vi "2010 Connection Lookup Tests.vi"(8 "error in":errorcluster) -> (0 "error out":errorcluster)   [LabVIEW 2020, in "Test_Routing Templates.lvlib"]
uses:
  Test_Routing Templates.lvlib
  <vilib>/addons/_JKI Toolkits/Caraya/classes/Test/Test.lvclass
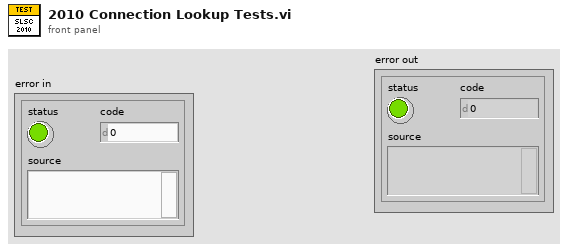
[diagram p1: front panel]
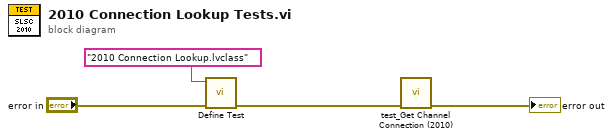
[diagram p0: block diagram]
diagram:
  n1 = call <vilib>:"Define Test.vi"("error in (no error)"="error in", "Label (VI Title)"="2010 Connection Lookup.lvclass") -> ("error out"=w2:errorcluster)  [unwired: 9 in]
  n2 = call "test_Get Channel Connection (2010).vi"("error in (no error)"=w2) -> ("error out"=→"error out":errorcluster)  [unwired: 10 in]
